vi "local.Initialize (Device).vi"(0 "devices":refnum<k21>, 7 "reservation access (Read/Write)":i32(ring)=3 items=["None"=0, "Read Only"=1, "Read/Write"=3], 9 "reservation group":string, 11 "error in (no error)":errorcluster, 12 "connect timeout (60 sec)":dbl=60.0) -> (4 "SLSC Local out":refnum<class "SLSC Interface.lvclass">, 15 "error out":errorcluster)   [LabVIEW 2016, in "SLSC Interface.lvclass"]
uses:
  SLSC Interface Class/SLSC Interface.lvclass
  <vilib>/SLSC/Initialize Session with Devices.vi
  SLSC Interface Class/Write session.vi
  <vilib>/SLSC/SLSC.lvlib
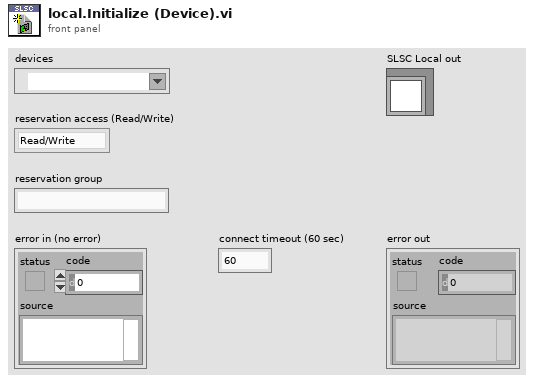
[diagram p1: front panel]
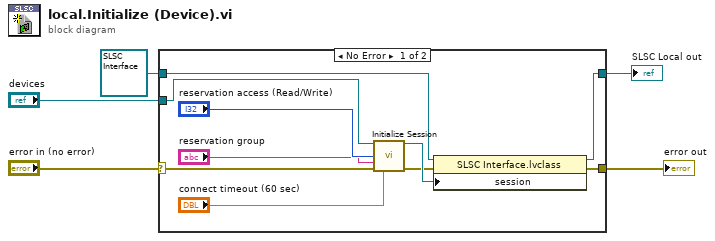
[diagram p0: block diagram]
diagram:
  n1 = case shown="No Error" "error in (no error)" {
    selector: "error in (no error)" -> [w15 w17]
    tunnel: [w6 w17] -> w4
    tunnel: [w9 w16] -> w3
    tunnel: refnum<class "SLSC Interface.lvclass"> refnum ("SLSC Interfaces.lvlib:SLSC Interface.lvclass") -> [w10 w16]
    tunnel: "devices" -> [w14 _]
    frame No Error {
      n2 = call-poly <vilib>:"Initialize Session.vi"("devices"=w14, "reservation access (Read/Write)"="reservation access (Read/Write)", "reservation group"="reservation group", "error in (no error)"=w15, "connect timeout (60 sec)"="connect timeout (60 sec)") -> ("session out"=w8:refnum<k21>, "error out"=w7:errorcluster)  [unwired: 9 in]
      n3 = property class="SLSC Interface.lvclass"(reference=w10, error in=w7, "session"=w8) -> (reference out=w9:refnum<class "SLSC Interface.lvclass">, error out=w6:errorcluster)
    }
    frame Error {
    }
  }
  "error out" <- w4
  "SLSC Local out" <- w3
